vi "Update Alarming Value.vi"(10 "Sample DBL":dbl, 11 "Virtual Sensor from CSV in":refnum<class "Virtual Sensor from CSV.lvclass">) -> (3 "Virtual Sensor from CSV out":refnum<class "Virtual Sensor from CSV.lvclass">)   [LabVIEW 2024, in "Virtual Sensor from CSV.lvclass"]
uses:
  Virtual Sensor from CSV.lvclass
  Virtual Sensor from CSV.lvclass/Virtual Sensor from CSV.ctl
  Action Point/Action Point.lvclass
  Alarming-Actor/Source/Alarming Actor/Alarming Actor Messages/Update Value Msg/Update Value Msg.lvclass
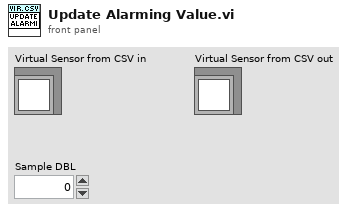
[diagram p1: front panel]
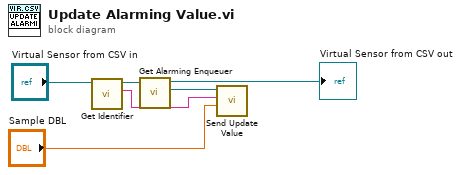
[diagram p0: block diagram]
diagram:
  n1 = call "Get Identifier.vi"("Action Point in"="Virtual Sensor from CSV in") -> ("Identifier"=w5:string, "Action Point out"=w4:refnum<class "Virtual Sensor from CSV.lvclass">)  [unwired: 9 in]
  n2 = call "Get Alarming Enqueuer.vi"("Action Point in"=w4) -> ("Alarming Enqueuer"=w3:refnum<class "Message Enqueuer.lvclass">, "Action Point out"=→"Virtual Sensor from CSV out":refnum<class "Virtual Sensor from CSV.lvclass">)  [unwired: 9 in]
  n3 = call "Send Update Value.vi"("Value"="Sample DBL", "Identifier"=w5, "Message Enqueuer"=w3) -> ()  [unwired: 7 in, 2 out]
